vi "wait on semaphores with timeout.vi"(8 "error in (no error)":errorcluster, 10 "abs sec timeout":dbl, 11 "semaphores in":T1[](array[typedef])) -> (0 "error out":errorcluster, 3 "semaphores out":T1[](array[typedef]))   [LabVIEW 2014, in "Shared Memory runtime.lvclass"]
uses:
  Shared Memory runtime.lvclass
  controls/semaphore data.ctl
  <vilib>/NI/NI Linux RT IPC/POSIX Threads/Classes/Semaphore/Controls/reference.ctl
  <vilib>/NI/NI Linux RT IPC/POSIX Threads/Classes/Semaphore/Semaphore.lvclass
  <vilib>/NI/NI Linux RT IPC/POSIX Threads/Classes/Semaphore/Public VIs/Semaphore Timed Wait (absolute seconds).vi
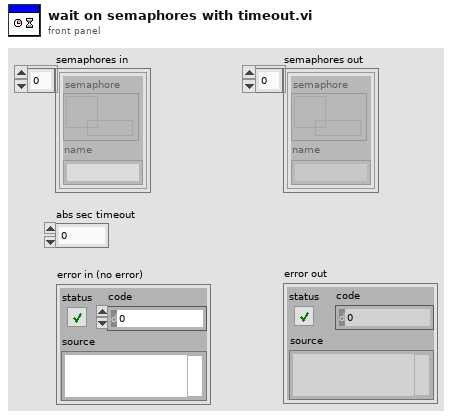
[diagram p1: front panel]
types:
  T1 = typedef "Shared Memory runtime.lvclass/semaphore data.ctl" = cluster{"semaphore":T2, "name":string}
  T2 = typedef "Linux RT IPC.POSIX Threads.lvlib/Semaphore.lvclass/reference.ctl" = refnum<data-value>
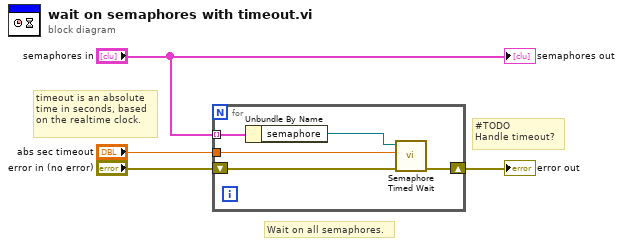
[diagram p0: block diagram]
diagram:
  # "timeout is an absolute time in seconds, based on the realtime clock."
  # "#TODO\nHandle timeout?"
  # "Wait on all semaphores."
  n1 = for {
    shift-right: [w8] -> w3
    shift-left: "error in (no error)" -> [w9]
    tunnel: "semaphores in" -> [w7] mode=indexing
    tunnel: "abs sec timeout" -> [w5]
    n2 = Unbundle By Name(w7) -> ("semaphore"=w6:T2)
    n3 = call-poly <vilib>:"Semaphore Timed Wait.vi"("error in (no error)"=w9, "absolute timeout (seconds)"=w5, "Semaphore in"=w6) -> ("error out"=w8:errorcluster)  [unwired: 6 in, 2 out]
  }
  "error out" <- w3
  "semaphores out" <- "semaphores in"
